vi "UHR-Fleezers Control (host) - Lorentz v2.vi"() -> ()   [LabVIEW 2014] (continued)
            n2219 = Build Cluster Array(w3307, w3324, w3323, w3322) -> (w3321:T46)
            n2220 = for {
              tunnel: w3343 -> [w3354]
              tunnel: w3321 -> [w3355] mode=indexing
              shift-right: [w3352] -> w3319
              shift-left: TRUE -> [w3353]
              shift-right: [w3351] -> w3317
              shift-left: _ -> [w3347]
              shift-right: [w3350] -> w3316
              shift-left: _ -> [w3346]
              shift-right: [w3349] -> w3315
              shift-left: _ -> [w3345]
              shift-right: [w3348] -> w3314
              shift-left: _ -> [w3344]
              n2221 = case shown="True" w3353 {
                selector: w3353 -> [w3360 _]
                tunnel: w3355 -> [_ w3369]
                tunnel: w3354 -> [_ w3367]
                tunnel: [w3360 w3365] -> w3352
                tunnel: [w3359 w3364] -> w3351
                tunnel: [w3358 w3363] -> w3350
                tunnel: [w3357 w3362] -> w3349
                tunnel: [w3356 w3361] -> w3348
                tunnel: w3347 -> [w3359 _]
                tunnel: w3346 -> [w3358 _]
                tunnel: w3345 -> [w3357 _]
                tunnel: w3344 -> [w3356 _]
                frame False {
                }
                frame True {
                  n2222 = Unbundle(w3369) -> (w3368:T45)
                  n2223 = call "isclickinwindow.vi"("Image Param"=w3368, "Point32"=w3367) -> ("4 Y"=w3361:i32, "3 Height"=w3362:i32, "2 X"=w3363:i32, "1 Width"=w3364:i32, "In image?"=w3366:bool)  [unwired: 1 in]
                  n2224 = Not(x=w3366) -> (.not. x?=w3365:bool)
                }
              }
            }
            n2225 = Not(x=w3319) -> (.not. x?=w3318:bool)
            n2226 = case shown="True" w3318 {
              tunnel: w3316 -> [_ w3383]
              tunnel: w3314 -> [_ w3382]
              tunnel: w3317 -> [_ w3381]
              tunnel: w3315 -> [_ w3380]
              frame False {
              }
              frame True {
                w3370 = FALSE ("Get Point")
                n2227 = local read "Scan lines (y)"() -> (w3385:u64)
                n2228 = disable-structure shown="Disabled" {
                  frame Disabled {
                  }
                  frame Enabled {
                  }
                }
                n2229 = local read "Actual MCL Inc (V)"() -> (w3379:dbl)
                n2230 = local read "Scan steps (MCL)"() -> (w3384:u64)
                n2231 = Divide "Y Pix/step"(x=w3380, y=w3385) -> (x/y=w3392:dbl)
                n2232 = Divide "Y V/pix"(x=w3379, y=w3392) -> (x/y=w3391:dbl)
                n2233 = Divide "Y half step offset"(x=w3379, y=2.0) -> (x/y=w3393:dbl)
                n2234 = Divide "X pix/step"(x=w3381, y=w3384) -> (x/y=w3390:dbl)
                n2235 = Negate(x=w3393) -> (-x=w3394:dbl)
                n2236 = local read "Initial Y"() -> (w3400:dbl)
                n2237 = Multiply(x=w3382, y=w3391) -> (x*y=w3401:dbl)
                n2238 = Divide "X half step offset"(x=w3379, y=2.0) -> (x/y=w3387:dbl)
                n2239 = Divide "X V/pix"(x=w3379, y=w3390) -> (x/y=w3389:dbl)
                n2240 = Multiply(x=w3379, y=w3384) -> (x*y=w3396:dbl)
                n2241 = Compound Arithmetic op=ADD(w3394, w3401, w3400) -> (w3371:dbl)
                "Pointer Y (V)" <- w3371
                n2242 = Multiply(x=w3389, y=w3383) -> (x*y=w3398:dbl)
                n2243 = Negate(x=w3387) -> (-x=w3386:dbl)
                n2244 = local read "Initial X"() -> (w3399:dbl)
                n2245 = Negate(x=w3398) -> (-x=w3397:dbl)
                n2246 = Compound Arithmetic op=ADD(w3386, w3396, w3399, w3397) -> (w3372:dbl)
                "Pointer X (V)" <- w3372
                n2247 = case shown="True" "Set High F Confocal Spot (X-Y)" {
                  tunnel: w3372 -> [_ w3402]
                  tunnel: w3371 -> [_ w3403]
                  frame False {
                  }
                  frame True {
                    "Confocal Y 2 (V)" <- w3403
                    "Confocal X 2 (V)" <- w3402
                  }
                }
                n2248 = Or(x="Set X Only", y="Set Confocal Spot (X-Y)") -> (x .or. y?=w3375:bool)
                n2249 = Or(x="Set Confocal Spot (X-Y)", y="Set Y Only") -> (x .or. y?=w3374:bool)
                n2250 = case shown="True" w3375 {
                  tunnel: w3372 -> [_ w3404]
                  frame False {
                  }
                  frame True {
                    n2251 = property on="AO2" class="Slide (strict)"("Val(Sgnl)"=w3404) -> ()  [unwired: 2 in, 2 out]
                    "Confocal X 1 (V)" <- w3404
                  }
                }
                n2252 = case shown="True" w3374 {
                  tunnel: w3371 -> [_ w3405]
                  frame False {
                  }
                  frame True {
                    n2253 = property on="AO1" class="Slide (strict)"("Val(Sgnl)"=w3405) -> ()  [unwired: 2 in, 2 out]
                    "Confocal Y 1 (V)" <- w3405
                  }
                }
                n2254 = local write "Set High F Confocal Spot (X-Y)"(w3370) -> ()
                n2255 = local write "Set Confocal Spot (X-Y)"(w3370) -> ()
                n2256 = local write "Set X Only"(w3370) -> ()
                n2257 = local write "Set Y Only"(w3370) -> ()
              }
            }
          }
          frame 3 {
            n2258 = local read "BD 2 Frequency 1 (MHz)"() -> (w3407:dbl)
            n2259 = local read "BD 1 Frequency 1 (MHz)"() -> (w3408:dbl)
            n2260 = local write "Manipulating Trap"(TRUE ("Manipulating Trap")) -> ()
            n2261 = local write "Coords"(T9 {"Horizontal"=0, "Vertical"=0} ("Coords")) -> ()
            n2262 = while {
              tunnel: w3412 -> [w3417]
              tunnel: w3410 -> [w3416]
              tunnel: w3408 -> [w3415]
              tunnel: w3407 -> [w3414]
              tunnel: w3406 -> [w3413]
              stop <- w3418 stop-if-true
              n2263 = event shown="[0] \"Pane\": Mouse Move" {
                selector: _ -> [_ _]
                dyn-events: _ -> [_ _]
                timeout: _ -> [_ _]
                tunnel: ["Force Manip Abort" w3482] -> w3418
                tunnel: w3417 -> [w3425 _]
                tunnel: w3416 -> [w3423 _]
                tunnel: w3415 -> [w3422 _]
                tunnel: w3414 -> [w3421 _]
                tunnel: w3413 -> [w3419 _]
                event Mouse Move {
                  n2264 = event-data() -> ("Time"=w3426:u32, "Coords"=w3427:T9)  [unwired: 3 out]
                  n2265 = Less?(x=w3426, y=w3425) -> (x < y?=w3424:bool)
                  n2266 = case "Makes sure old motion events prior to mouse click aren't used" shown="False" w3424 {
                    tunnel: w3427 -> [w3469 _]
                    tunnel: w3423 -> [w3470 _]
                    tunnel: w3422 -> [w3444 _]
                    tunnel: w3421 -> [w3443 _]
                    tunnel: w3419 -> [w3428 _]
                    frame False {
                      n2267 = Subtract(x=w3469, y=w3470) -> (x-y=w3468:T9)
                      "Coords" <- w3468
                      n2268 = local read "Y RF Frequency Limits (MHz)"() -> (w3429:T20)
                      n2269 = To Double Precision Float(number=w3468) -> (double precision float=w3467:cluster{"Horizontal":dbl, "Vertical":dbl})
                      n2270 = Multiply(x=cluster{"Horizontal":dbl, "Vertical":dbl} {"Horizontal"=-1.0, "Vertical"=1.0}, y="Manipulation Scaling") -> (x*y=w3463:cluster{"Horizontal":dbl, "Vertical":dbl})
                      n2271 = local read "X RF Frequency Limits (MHz)"() -> (w3430:T20)
                      n2272 = Multiply(x=w3467, y=w3463) -> (x*y=w3465:cluster{"Horizontal":dbl, "Vertical":dbl})
                      n2273 = Unbundle By Name(w3465) -> ("Horizontal"=w3460:dbl, "Vertical"=w3464:dbl)
                      n2274 = Unbundle By Name(w3429) -> ("Maximum"=w3432:dbl, "Minimum"=w3431:dbl)
                      n2275 = Boolean To (0,1)(Boolean="Manip. X?") -> (0, 1=w3458:i16)
                      n2276 = Boolean To (0,1)(Boolean="Manip. Y?") -> (0, 1=w3455:i16)
                      n2277 = local read "BD 1 Frequency 2 (MHz)"() -> (w3446:dbl)
                      n2278 = Multiply(x=w3464, y=w3455) -> (x*y=w3457:dbl)
                      n2279 = Multiply(x=w3458, y=w3460) -> (x*y=w3461:dbl)
                      n2280 = local read "BD 2 Frequency 2 (MHz)"() -> (w3445:dbl)
                      n2281 = Unbundle By Name(w3430) -> ("Maximum"=w3434:dbl, "Minimum"=w3433:dbl)
                      n2282 = Add(x=w3443, y=w3457) -> (x+y=w3436:dbl)
                      n2283 = Add(x=w3444, y=w3461) -> (x+y=w3438:dbl)
                      n2284 = In Range and Coerce(upper limit=w3434, x=w3438, lower limit=w3433) -> (coerced(x)=w3437:dbl)  [unwired: 1 out]
                      n2285 = In Range and Coerce(upper limit=w3432, x=w3436, lower limit=w3431) -> (coerced(x)=w3435:dbl)  [unwired: 1 out]
                      n2286 = Subtract(x=w3437, y=w3446) -> (x-y=w3454:dbl)
                      n2287 = Subtract(x=w3435, y=w3445) -> (x-y=w3453:dbl)
                      n2288 = Square(x=w3454) -> (x^2=w3452:dbl)
                      n2289 = Square(x=w3453) -> (x^2=w3451:dbl)
                      n2290 = Add(x=w3452, y=w3451) -> (x+y=w3450:dbl)
                      n2291 = Square Root(x=w3450) -> (sqrt(x)=w3447:dbl)
                      n2292 = In Range and Coerce(upper limit="Limit Max (MHz)", x=w3447, lower limit="Limit Min (MHz)") -> (In Range?=w3440:bool)  [unwired: 1 out]
                      n2293 = Not(x="Limits Enable") -> (.not. x?=w3439:bool)
                      n2294 = Or(x=w3440, y=w3439) -> (x .or. y?=w3441:bool)
                      n2295 = case shown="True" w3441 {
                        tunnel: w3447 -> [_ w3472]
                        tunnel: w3437 -> [_ w3479]
                        tunnel: w3446 -> [_ w3478]
                        tunnel: w3435 -> [_ w3477]
                        tunnel: w3445 -> [_ w3476]
                        tunnel: w3430 -> [_ w3474]
                        tunnel: w3429 -> [_ w3473]
                        tunnel: w3428 -> [_ w3471]
                        frame False {
                        }
                        frame True {
                          n2296 = local read "BD 1 Frequency 3 (MHz)"() -> (w3480:dbl)
                          n2297 = local read "BD 2 Frequency 3 (MHz)"() -> (w3475:dbl)
                          n2298 = local write "Trap Delta (MHz)"(w3472) -> ()
                          n2299 = call "set RF board frequency - interlace.vi"("Board 2 Frequency Limits"=w3473, "Board 1 Frequency Limits"=w3474, "FPGA VI Reference In"=w3471, "Board 2 Frequency 3 (MHz)"=w3475, "Board 1 Frequency 3 (MHz)"=w3480, "Board 2 Frequency 2 (MHz)"=w3476, "Board 2 Frequency 1 (MHz)"=w3477, "Board 1 Frequency 2 (MHz)"=w3478, "Board 1 Frequency 1  (MHz)"=w3479) -> ()  [unwired: 1 in, 2 out]
                          n2300 = local write "BD 2 Frequency 1 (MHz)"(w3477) -> ()
                          n2301 = local write "BD 1 Frequency 1 (MHz)"(w3479) -> ()
                        }
                      }
                    }
                    frame True {
                    }
                  }
                }
                event Mouse Up {
                  n2302 = event-data() -> ("Button"=w3481:u16)  [unwired: 8 out]
                  n2303 = case shown="3" w3481 {
                    tunnel: [FALSE TRUE] -> w3482
                    frame 0, Default {
                    }
                    frame 3 {
                      n2304 = local read "Trap Delta (MHz)"() -> (w3484:dbl)
                      n2305 = property on="Initial delta (MHz)" class="DigNum (strict)"("Val(Sgnl)"=w3484) -> ()  [unwired: 2 in, 2 out]
                      n2306 = local write "Manipulating Trap"(FALSE ("Manipulating Trap")) -> ()
                    }
                  }
                }
              }
            }
          }
        }
      }
      event Timeout {
        n2307 = event-data() -> ()  [unwired: 4 out]
      }
      event "Stop All": Mouse Down {
        n2308 = event-data() -> ()  [unwired: 9 out]
      }
      event Mouse Move {
        n2309 = event-data() -> ()  [unwired: 6 out]
      }
    }
    n2310 = node-c288() -> ()  [unwired: 2 out]
  }
  n2311 = disable-structure shown="Disabled" {
    frame Disabled {
      n2312 = flat-sequence "Video" {
        tunnel: [w3499] -> w3488
        tunnel: w3488 -> [w3540]
        frame #0 {
          w3489 = FALSE ("File open?")
          n2313 = while {
            stop <- w3491 continue-if-true
            n2314 = call "Close Video Capture.vi"() -> ("error code OUT"=w3493:i32)
            n2315 = Equal?(x=w3493, y=0) -> (x = y?=w3491:bool)
          }
          n2316 = local write "New Video File"(w3489) -> ()
          n2317 = local write "File open?"(w3489) -> ()
          n2318 = local write "Save Video"(w3489) -> ()
          n2319 = local write "Stop All"(FALSE ("Stop All")) -> ()
        }
        frame #1 {
          n2320 = call "DMR_Init.vi"() -> ()  [unwired: 3 out]
        }
        frame #2 {
          w3494 = "DE245428202"  # MSU fleezers card #
          (unwired) "DE019116701"  # Illinois fleezers card #
          # "Setting the destination format to Mono8 makes sure that the image can be displayed in the intensity plot."
          n2321 = call "DMR_GetDevice.vi"("search string IN"=w3494) -> ("device handle OUT"=w3517:i32)  [unwired: 4 in, 2 out]
          n2322 = call "DMR_OpenDevice.vi"("device handle IN"=w3517) -> ("driver handle OUT"=w3500:i32)  [unwired: 4 out]
          n2323 = call "DMR_FindList.vi"("flags IN"=u32 0 ("flags"), "list name IN"="" ("String"), "list type IN"=T47."camera descriptions", "driver handle IN"=w3500) -> ("list handle OUT"=w3503:i32)  [unwired: 2 out]
          n2324 = call "DMR_FindList.vi"("flags IN"=u32 0 ("flags"), "list name IN"="Base", "list type IN"=T47."setting", "driver handle IN"=w3500) -> ("list handle OUT"=w3501:i32)  [unwired: 2 out]
          n2325 = call "OBJ_GetHandle.vi"("object name IN"="VideoStandard", "list handle IN"=w3503) -> ("object handle OUT"=w3497:i32)  [unwired: 3 out]
          n2326 = call "OBJ_GetHandle.vi"("object name IN"="PixelFormat", "list handle IN"=w3501) -> ("object handle OUT"=w3511:i32)  [unwired: 3 out]
          n2327 = call "OBJ_SetS.vi"("value index IN"=0, "value IN"="NTSC M", "object handle IN"=w3497) -> ()  [unwired: 2 out]
          n2328 = call "OBJ_SetS.vi"("value index IN"=0, "value IN"="Mono8" ("value"), "object handle IN"=w3511) -> ()  [unwired: 2 out]
          n2329 = call "OBJ_GetHandle.vi"("object name IN"="VideoChannel", "list handle IN"=w3501) -> ("object handle OUT"=w3507:i32)  [unwired: 3 out]
          n2330 = while {
            tunnel: [w3521] -> w3499
            tunnel: w3500 -> [w3518]
            stop <- w3519 continue-if-true
            n2331 = call "DMR_ImageRequestSingle.vi"("request control IN"=0, "driver handle IN"=w3518) -> ("error code OUT"=w3520:i32, "driver handle OUT"=w3521:i32)  [unwired: 2 out]
            n2332 = Equal To 0?(x=w3520) -> (x = 0?=w3519:bool)
          }
          n2333 = call "OBJ_SetI.vi"("value index IN"=0, "value IN"="Video channel", "object handle IN"=w3507) -> ()  [unwired: 2 out]
        }
        frame #3 {
          w3528 = T25 0 items=["Grayscale (U8)", "Grayscale (I16)", "Grayscale (SGL)", "Complex (CSG)", "RGB (U32)", "HSL (U32)", "RGB (U64)"] ("Image Type")
          w3536 = T25 0 items=["Grayscale (U8)", "Grayscale (I16)", "Grayscale (SGL)", "Complex (CSG)", "RGB (U32)", "HSL (U32)", "RGB (U64)"] ("Image Type")
          n2334 = call "IMAQ AVI2 Get Codec Names"() -> ("Codec Names"=w3523:string[])  [unwired: 10 in, 1 out]
          "Installed Codec Names" <- w3523
          n2335 = for "Create Greyscale map" {
            N: 256 -> [_]
            tunnel: [w3542] -> w3525 mode=indexing
            workers-P: _ -> [_]
            i -> [w3545]
            n2336 = To Unsigned Byte Integer(number=w3545) -> (unsigned 8bit integer=w3541:u8)
            n2337 = Join Numbers(hi=w3541, lo=w3541) -> ((hi.lo)=w3544:u16)
            n2338 = Join Numbers(hi=w3541, lo=w3541) -> ((hi.lo)=w3543:u16)
            n2339 = Join Numbers(hi=w3544, lo=w3543) -> ((hi.lo)=w3542:u32)
          }
          n2340 = property on="Codec choice" class="CmbBox"("Strings[]"=w3523) -> ()  [unwired: 2 in, 2 out]
          n2341 = call "IMAQ Create"("Image Name"="Scaled video", "Image Type"=w3528) -> ("New Image"=w3527:T2)  [unwired: 2 in, 2 out]
          n2342 = call "IMAQ Create"("Image Name"="Main video", "Image Type"=w3536) -> ("New Image"=w3537:T2)  [unwired: 2 in, 2 out]
          n2343 = node-c288(0 ("Processor")) -> (w3535:T35)  [unwired: 3 out]
          n2344 = Initialize Array(u32 0 ("Window Number (0...15)"), 480 ("dimension size"), 640 ("dimension size")) -> (w3530:u32[][])
          n2345 = timed-loop {
            tunnel: w3540 -> [w3562]
            tunnel: [w3561] -> w3539
            tunnel: w3537 -> [w3560]
            timing: w3535 -> [_]
            timing-out: [_] -> w3534
            tunnel: w3530 -> [w3553]
            tunnel: w3527 -> [w3551]
            tunnel: w3525 -> [w3550]
            stop <- w3552 stop-if-true
            # "This block performs the \nactual image capture."
            n2346 = node-c288() -> (→"Finished Late? [i-1]":bool)  [unwired: 5 out]
            n2347 = local read "Stop All"() -> (w3552:bool)
            n2348 = feedback #1(T48 refnum ("AVI Refnum")) -> (w3558:T48)
            n2349 = case shown="True" "New Video File" {
              tunnel: [w3575 w3576] -> w3549
              tunnel: w3558 -> [w3575 w3577]
              frame False {
              }
              frame True {
                n2350 = flat-sequence {
                  tunnel: w3577 -> [w3579]
                  tunnel: [w3581] -> w3576
                  frame #0 {
                    n2351 = local read "File open?"() -> (w3578:bool)
                    n2352 = case shown="True" w3578 {
                      tunnel: w3579 -> [_ w3580]
                      frame False {
                      }
                      frame True {
                        n2353 = call "IMAQ AVI2 Close"("AVI Refnum"=w3580) -> ()  [unwired: 10 in, 1 out]
                      }
                    }
                  }
                  frame #1 {
                    n2354 = local write "New Video File"(FALSE ("New Video File")) -> ()
                    n2355 = call "Create new save file.vi"("Ext"=".avi" ("string"), "Index In"="Video Index") -> ("Path Out"=w3584:path, "Index Out"=w3586:dbl)  [unwired: 1 in]
                    "Path Out" <- w3584
                    n2356 = local write "Video Index"(w3586) -> ()
                    n2357 = call "IMAQ AVI2 Create"("Codec"="Codec choice", "Frames Per Second"=u32 30, "AVI Path"=w3584) -> ("AVI Refnum"=w3581:T48)  [unwired: 7 in, 1 out]
                    "File open?" <- TRUE ("Files open?")
                  }
                }
              }
            }
            n2358 = feedback-in #1(w3549) -> ()
            n2359 = call "DMR_ImageRequestWaitFor.vi"("queue number IN"=0, "timeout(ms) IN"=500, "driver handle IN"=w3562) -> ("error code OUT"=w3566:i32, "request number OUT"=w3563:i32, "driver handle OUT"=w3564:i32)
            n2360 = Equal To 0?(x=w3566) -> (x = 0?=w3565:bool)
            n2361 = Reciprocal(x="Video Capture Rate (Hz)") -> (1/x=w3556:dbl)
            n2362 = Multiply(x=w3556, y=1000.0) -> (x*y=w3554:dbl)
            n2363 = case shown="True" w3565 {
              tunnel: w3564 -> [w3590 w3627]
              tunnel: w3563 -> [_ w3626]
              tunnel: [w3590 w3623] -> w3561
              tunnel: w3560 -> [_ w3609]
              tunnel: w3553 -> [_ w3612]
              tunnel: w3549 -> [_ w3592]
              tunnel: w3551 -> [_ w3606]
              tunnel: w3550 -> [_ w3605]
              frame False {
              }
              frame True {
                w3617 = u32 0 ("X-offset IN")
                n2364 = call "DMR_GetImageRequestBufferData.vi"("driver handle IN"=w3627, "request number IN"=w3626) -> ("width OUT"=w3616:i32, "height OUT"=w3615:i32, "driver handle OUT"=w3622:i32, "request number OUT"=w3621:i32, "bytes per pixel OUT"=w3618:i32)  [unwired: 13 out]
                n2365 = call "DMR_GetImageRequestBufferImageData.vi"("driver handle IN"=w3622, "request number IN"=w3621, "bytes per pixel IN"=w3618, "X-offset IN"=w3617, "Y-offset IN"=w3617, "height IN"=w3615, "width IN"=w3616) -> ("driver handle OUT"=w3620:u32, "request number OUT"=w3619:u32, "image OUT"=w3598:u32[][])  [unwired: 10 out]
                n2366 = Transpose 2D Array(2D array=w3598) -> (transposed array=w3604:u32[][])
                n2367 = Select(t=w3604, s="Flip Y (or X)", f=w3598) -> (s? t:f=w3603:u32[][])
                n2368 = call "DMR_ImageRequestUnlock.vi"("request number IN"=w3619, "driver handle IN"=w3620) -> ("driver handle OUT"=w3625:i32)  [unwired: 1 in, 2 out]
                n2369 = for {
                  tunnel: w3603 -> [w3662] mode=indexing
                  tunnel: [w3661] -> w3601 mode=indexing
                  n2370 = Reverse 1D Array(array=w3662) -> (reversed array=w3661:u32[])
                }
                n2371 = call "DMR_ImageRequestSingle.vi"("request control IN"=0, "driver handle IN"=w3625) -> ("driver handle OUT"=w3623:i32)  [unwired: 3 out]
                n2372 = Transpose 2D Array(2D array=w3601) -> (transposed array=w3602:u32[][])
                n2373 = Select(t=w3602, s="Flip Y (or X)", f=w3601) -> (s? t:f=w3599:u32[][])
                n2374 = Select(t=w3599, s="Flip Image", f=w3598) -> (s? t:f=w3596:u32[][])
                n2375 = case shown="True" "Averaging" {
                  tunnel: w3596 -> [w3673 w3678]
                  tunnel: [w3673 w3677] -> w3610
                  tunnel: w3612 -> [_ w3675]
                  frame False {
                  }
                  frame True {
                    (unwired) 1
                    w3683 = 1
                    n2376 = feedback #2(w3675) -> (w3674:u32[][])
                    n2377 = Add(x=w3678, y=w3674) -> (x+y=w3679:u32[][])
                    n2378 = Select(t=w3675, s="Reset Averaging", f=w3679) -> (s? t:f=w3681:u32[][])
                    n2379 = feedback-in #2(w3681) -> ()
                    n2380 = feedback #3(w3683) -> (w3676:i32)
                    n2381 = Divide(x=w3679, y=w3676) -> (x/y=w3680:dbl[][])
                    n2382 = Increment(x=w3676) -> (x+1=w3684:i32)
                    n2383 = To Unsigned Long Integer(number=w3680) -> (unsigned 32bit integer=w3677:u32[][])
                    n2384 = Select(t=w3683, s="Reset Averaging", f=w3684) -> (s? t:f=w3682:i32)
                    n2385 = feedback-in #3(w3682) -> ()
                  }
                }
                n2386 = case shown="True" "Zoom video window" {
                  tunnel: w3610 -> [_ w3641]
                  tunnel: w3606 -> [_ w3640]
                  frame False {
                  }
                  frame True {
                    n2387 = To Double Precision Float(number=w3641) -> (double precision float=w3638:dbl[][])
                    n2388 = In Range and Coerce(upper limit="Intensity Upper", x=w3638, lower limit="Intensity Lower") -> (coerced(x)=w3637:dbl[][])  [unwired: 1 out]
                    n2389 = Subtract(x="Intensity Upper", y="Intensity Lower") -> (x-y=w3634:dbl)
                    n2390 = Subtract(x=w3637, y="Intensity Lower") -> (x-y=w3635:dbl[][])
                    n2391 = Divide(x=w3635, y=w3634) -> (x/y=w3636:dbl[][])
                    n2392 = Multiply(x=255.0, y=w3636) -> (x*y=w3632:dbl[][])
                    n2393 = To Unsigned Byte Integer(number=w3632) -> (unsigned 8bit integer=w3639:u8[][])
                    n2394 = call "IMAQ ArrayToImage"("Image Pixels (U8)"=w3639, "Image"=w3640) -> ("Image Out"=w3628:T2)  [unwired: 4 in, 5 out]
                    n2395 = First Call?() -> (First Call?: T/F=w3629:bool)
                    n2396 = case shown="True" w3629 {
                      tunnel: w3628 -> [w3642 w3653]
                      frame False {
                        n2397 = flat-sequence {
                          tunnel: w3642 -> [w3648]
                          frame #0 {
                            w3645 = FALSE ("Get/Set Status? (Set)")
                            w3644 = 0 ("Window Number (0...15)")
                            n2398 = call "IMAQ WindSize"("Get/Set Status? (Set)"=w3645, "Window Number"=w3644) -> ("Width & Height out"=→"Window Size":cluster{"Width":i32, "Height":i32})  [unwired: 4 in, 2 out]
                            n2399 = call "IMAQ WindMove"("Window Number (0...15)"=w3644, "Get/Set Status? (Set)"=w3645) -> ("Coordinates (screen)"=→"Window Position":cluster{"X Position":i32, "Y Position":i32})  [unwired: 3 in, 1 out]
                            n2400 = call "IMAQ WindDraw"("Resize to Image Size? (Y)"=FALSE, "Window Number (0...15)"=w3644, "Image"=w3648) -> ()  [unwired: 7 in, 2 out]
                          }
                          frame #1 {
                            n2401 = call "IMAQ WindZoom 2"("Center Point"="Center Point", "Zoom to Fit? (False)"=FALSE, "Zoom Factor"="Zoom Factor") -> ()  [unwired: 5 in, 4 out]
                          }
                        }
                      }
                      frame True {
                        n2402 = flat-sequence {
                          tunnel: w3653 -> [w3656]
                          tunnel: [w3654] -> w3652
                          tunnel: w3652 -> [w3658]
                          frame #0 {
                            w3655 = TRUE ("Resize to Image Size? (Y)")
                            w3654 = 0 ("Window Number (0...15)")
                            n2403 = call "IMAQ WindNonTearing"("Window Number"=w3654, "NonTearing? (True)"=w3655) -> ()  [unwired: 8 in, 2 out]
                            n2404 = call "IMAQ WindDraw"("Resize to Image Size? (Y)"=w3655, "Window Number (0...15)"=w3654, "Image"=w3656) -> ()  [unwired: 7 in, 2 out]
                          }
                          frame #1 {
                            n2405 = call "IMAQ WindSize"("Scrollbars? (N)"=FALSE, "Width & Height"="Initial Window Size", "Window Number"=w3658) -> ()  [unwired: 3 in, 3 out]
                            n2406 = call "IMAQ WindMove"("Window Number (0...15)"=w3658, "Coordinates (screen)"="Initial Window Position") -> ()  [unwired: 3 in, 2 out]
                          }
                        }
                      }
                    }
                  }
                }
                n2407 = To Unsigned Byte Integer(number=w3610) -> (unsigned 8bit integer=w3608:u8[][])
                n2408 = call "IMAQ ArrayToImage"("Image Pixels (U8)"=w3608, "Image"=w3609) -> ("Image Out"=w3607:T2)  [unwired: 4 in, 5 out]
                "Primary Video Display" <- w3607
                n2409 = Not(x="Close Video File") -> (.not. x?=w3594:bool)
                n2410 = And(x="Save Video", y=w3594) -> (x .and. y?=w3591:bool)
                n2411 = case shown="True" "Save Image" {
                  tunnel: w3608 -> [_ w3687]
                  tunnel: w3605 -> [_ w3686]
                  frame False {
                  }
                  frame True {
                    n2412 = call <vilib>:"Flatten Pixmap.vi"("colors"=w3686, "8-bit pixmap"=w3687) -> ("image data"=w3693:T49)  [unwired: 4 in, 5 out]
                    n2413 = call "Create new save file.vi"("Insert"="video_frame_" ("string"), "Ext"=".bmp" ("string"), "Index In"="Image Index") -> ("Path Out"=w3689:path, "Index Out"=w3694:dbl)
                    n2414 = Increment(x=w3694) -> (x+1=w3688:dbl)
                    n2415 = local write "Image Index"(w3688) -> ()
                    n2416 = call <vilib>:"Write BMP File.vi"("image data"=w3693, "path to BMP file"=w3689) -> ()  [unwired: 1 in, 9 out]
                  }
                }
                n2417 = case shown="True" w3591 {
                  tunnel: w3592 -> [w3664 w3669]
                  tunnel: w3607 -> [_ w3668]
                  tunnel: "Close Video File" -> [w3663 _]
                  frame False {
                    n2418 = case shown="True" w3663 {
                      tunnel: w3664 -> [_ w3665]
                      frame False {
                      }
                      frame True {
                        w3666 = FALSE ("Save Video")
                        n2419 = call "IMAQ AVI2 Close"("AVI Refnum"=w3665) -> ()  [unwired: 10 in, 1 out]
                        n2420 = local write "File open?"(w3666) -> ()
                        n2421 = local write "Save Video"(w3666) -> ()
                      }
                    }
                  }
                  frame True {
                    n2422 = local read "File open?"() -> (w3667:bool)
                    n2423 = case shown="True" w3667 {
                      tunnel: w3669 -> [_ w3672]
                      tunnel: w3668 -> [_ w3671]
                      frame False {
                        n2424 = local write "New Video File"(TRUE ("New Video File")) -> ()
                      }
                      frame True {
                        n2425 = call "IMAQ AVI2 Write Frame"("Image"=w3671, "AVI Refnum"=w3672) -> ()  [unwired: 7 in, 3 out]
                      }
                    }
                  }
                }
              }
            }
            n2426 = node-c288(w3554, "Deadline (ms)") -> ()  [unwired: 1 out]
          }
          n2427 = node-c288(w3534) -> ()  [unwired: 1 out]
          n2428 = call "DMR_CloseDevice.vi"("driver handle IN"=w3539) -> ()  [unwired: 1 in, 4 out]
        }
        frame #4 {
          n2429 = call "DMR_Close.vi"() -> ()  [unwired: 1 out]
        }
      }
    }
    frame Enabled {
    }
  }
  n2430 = node-c288(3 ("Processor")) -> (w60:T35)  [unwired: 3 out]
  n2431 = timed-loop "Oscillate Trap/AOM (fishing, conjugate plane alignment)" {
    tunnel: [w3701] -> w65
    timing: w60 -> [_]
    timing-out: [_] -> w59
    tunnel: w21 -> [w3700]
    tunnel: w9 -> [w3699]
    stop <- w3701 stop-if-true
    n2432 = node-c288() -> ()  [unwired: 2 out]
    n2433 = event shown="[1] \"Fl. Triggered...\": Value Change" {
      selector: _ -> [_ _ _ _]
      dyn-events: _ -> [_ _ _ _]
      timeout: _ -> [_ _ _ _]
      tunnel: [FALSE ("Stop All") _ _ w4372] -> w3701
      tunnel: w3700 -> [w3704 _ _ _]
      tunnel: w3699 -> [_ _ w4309 _]
      event "Oscillate Set 1", "Fish for Tether": Value Change {
        n2434 = event-data() -> ()  [unwired: 6 out]
        n2435 = local read "Oscillate Set 1"() -> (w3708:bool)
        n2436 = Or(x=w3708, y="Fish for Tether") -> (x .or. y?=w3706:bool)
        n2437 = case shown="True" w3706 {
          tunnel: "Fish for Tether" -> [_ w3711]
          tunnel: w3704 -> [_ w3709]
          frame False {
          }
          frame True {
            n2438 = case shown="True" w3711 {
              selector: w3711 -> [w3714 w3720]
              tunnel: [w3714 w3720] -> w3710
              frame False {
              }
              frame True {
                n2439 = local write "Scan axis 2"(TRUE) -> ()
                n2440 = local write "Tether"(FALSE ("Tether")) -> ()
                n2441 = local read "Flow ON during cal?"() -> (w3715:bool)
                n2442 = property on="Trap Delta (MHz)" class="DigNum (strict)"("Val(Sgnl)"="Furthest Delta (MHz)") -> ()  [unwired: 2 in, 2 out]
                n2443 = Or(x="Flow ON during \nfishing?", y=w3715) -> (x .or. y?=w3716:bool)
                n2444 = Wait (ms)(milliseconds to wait=u32 500) -> ()  [unwired: 1 out]
                n2445 = property on="Sample Channel\nFlow" class="Bool (strict)"("Val(Sgnl)"=w3716) -> ()  [unwired: 2 in, 2 out]
              }
            }
            n2446 = node-c288() -> (w3713:T35)  [unwired: 1 in, 3 out]
            n2447 = timed-loop "Oscillate AOD" {
              timing: w3713 -> [_]
              timing-out: [_] -> w3712
              tunnel: w3710 -> [w3724]
              tunnel: w3709 -> [w3723]
              i -> [w3732]
              stop <- w3730 stop-if-true
              n2448 = node-c288() -> (w3731:i64)  [unwired: 1 out]
              n2449 = flat-sequence {
                tunnel: w3732 -> [w3759]
                tunnel: w3731 -> [w3758]
                tunnel: w3724 -> [w3742]
                tunnel: [w3742] -> w3729
                tunnel: [w3741] -> w3728
                tunnel: [w3740] -> w3727
                tunnel: [w3737] -> w3725
                tunnel: w3723 -> [w3733]
                tunnel: w3729 -> [w3806]
                tunnel: w3728 -> [w3804]
                tunnel: w3727 -> [w3803]
                tunnel: [w3802] -> w3726
                tunnel: w3725 -> [w3801]
                tunnel: [w3878] -> w3730
                tunnel: w3726 -> [w3877]
                frame #0 {
                  # "w (rad/s)"
                  # "t (s)"
                  n2450 = Divide(x=w3758, y=i64 1000) -> (x/y=w3734:dbl)
                  n2451 = local read "BD 1 Frequency 2 (MHz)"() -> (w3736:dbl)
                  n2452 = Multiply(x="Osc. freq. (Hz)", y=6.283185307179586) -> (x*y=w3756:dbl)
                  n2453 = Multiply(x=w3734, y=w3759) -> (x*y=w3755:dbl)
                  n2454 = Multiply(x=w3756, y=w3755) -> (x*y=w3739:dbl)
                  n2455 = local read "BD 1 Frequency 1 (MHz)"() -> (w3744:dbl)
                  n2456 = case shown="True" w3742 {
                    tunnel: w3739 -> [w3765 w3784]
                    tunnel: w3744 -> [_ w3792]
                    tunnel: w3736 -> [_ w3793]
                    tunnel: [w3762 w3788] -> w3735
                    tunnel: [FALSE w3766] -> w3740
                    tunnel: [0.0 w3780] -> w3737
                    frame False {
                      n2457 = Sine(x=w3765) -> (sin(x)=w3763:dbl)
                      n2458 = Multiply(x=w3763, y="Osc. amp. (MHz)") -> (x*y=w3762:dbl)
                    }
                    frame True {
                      # "trap position goes from 0 to 1 (0 is when it is furthest away, 1 is when closest)\nso we want to test for tether only when farther away, or x < 1"
                      # "quit if taking too long"
                      # "oscillate the trap"
                      # "Test for tether"
                      n2459 = local read "Vec Mean of T1 T2"() -> (w3769:dbl[])
                      "Trigger Signal" <- w3769
                      n2460 = Cosine(x=w3784) -> (cos(x)=w3796:dbl)
                      n2461 = Subtract(x=w3793, y=w3792) -> (x-y=w3791:dbl)
                      n2462 = Decrement(x=w3796) -> (x-1=w3795:dbl)
                      n2463 = Subtract(x=w3791, y="Closest Delta (MHz)") -> (x-y=w3789:dbl)
                      n2464 = Divide(x=w3795, y=-2.0) -> (x/y=w3779:dbl)
                      n2465 = Greater?(x=w3769, y="Stop F (pN)") -> (0:w3786:bool[])
                      n2466 = Multiply(x=w3779, y=w3789) -> (x*y=w3788:dbl)
                      n2467 = Less?(x=w3779, y="Fish mask thresh") -> (x < y?=w3778:bool)
                      n2468 = Boolean To (0,1)(Boolean=w3778) -> (0, 1=w3776:i16)
                      n2469 = Multiply(x=w3776, y=w3769) -> (x*y=w3775:dbl[])
                      n2470 = Divide(x=w3784, y=6.283185307179586) -> (x/y=w3783:dbl)
                      n2471 = Round Toward +Infinity(x=w3783) -> (ceil(x): smallest int >= x=w3780:dbl)
                      "Attempts" <- w3780
                      n2472 = Greater?(x=w3775, y="Stop F (pN) (mask)") -> (0:w3773:bool[])
                      n2473 = Or Array Elements(Boolean array=w3786) -> (logical OR=w3771:bool)
                      n2474 = Or Array Elements(Boolean array=w3773) -> (logical OR=w3770:bool)
                      n2475 = Greater?(x=w3780, y="Attempt Limit") -> (0:w3782:bool)
                      n2476 = case shown="True" w3782 {
                        frame False {
                        }
                        frame True {
                          n2477 = local write "Fish for Tether"(FALSE ("Fish for Tether")) -> ()
                          n2478 = call <vilib>:"Beep.vi"() -> ()  [unwired: 3 in, 9 out]
                          n2479 = local read "Messages"() -> (w3798:string)
                          n2480 = call "Update messages.vi"("Message to add"="Tether fishing timeout." ("Messages"), "Old message string"=w3798) -> ("New message string"=→"Messages":string)
                        }
                      }
                      n2481 = Select(t=w3771, s="Normal (on) or masked test (off)", f=w3770) -> (s? t:f=w3768:bool)
                      n2482 = And(x="Stop Fishing When Tether", y=w3768) -> (x .and. y?=w3766:bool)
                    }
                  }
                  n2483 = local read "BD 2 Frequency 1 (MHz)"() -> (w3743:dbl)
                  n2484 = Select(t=w3744, s="Scan axis 2", f=w3743) -> (s? t:f=w3747:dbl)
                  n2485 = Add(x=w3735, y=w3747) -> (x+y=w3741:dbl)
                  n2486 = Select(t=w3741, s="Scan axis 2", f=w3744) -> (s? t:f=w3750:dbl)
                  n2487 = Select(t=w3743, s="Scan axis 2", f=w3741) -> (s? t:f=w3749:dbl)
                  n2488 = local read "BD 2 Frequency 2 (MHz)"() -> (w3752:dbl)
                  n2489 = local read "BD 2 Frequency 3 (MHz)"() -> (w3751:dbl)
                  n2490 = local read "Y RF Frequency Limits (MHz)"() -> (w3745:T20)
                  n2491 = local read "X RF Frequency Limits (MHz)"() -> (w3746:T20)
                  n2492 = local read "BD 1 Frequency 3 (MHz)"() -> (w3753:dbl)
                  n2493 = call "set RF board frequency - interlace.vi"("Board 2 Frequency Limits"=w3745, "Board 1 Frequency Limits"=w3746, "FPGA VI Reference In"=w3733, "Board 2 Frequency 3 (MHz)"=w3751, "Board 1 Frequency 3 (MHz)"=w3753, "Board 2 Frequency 2 (MHz)"=w3752, "Board 2 Frequency 1 (MHz)"=w3749, "Board 1 Frequency 2 (MHz)"=w3736, "Board 1 Frequency 1  (MHz)"=w3750) -> ()  [unwired: 1 in, 2 out]
                }
                frame #1 {
                  n2494 = And(x=w3806, y=w3803) -> (x .and. y?=w3805:bool)
                  n2495 = case "Only if were fishing and now formed tether" shown="True" w3805 {
                    tunnel: w3804 -> [w3808 w3823]
                    tunnel: [w3807 w3822] -> w3802
                    tunnel: w3801 -> [_ w3818]
                    frame False {
                      n2496 = local read "Fish for Tether"() -> (w3807:bool)
                      n2497 = case shown="False" w3807 {
                        tunnel: w3808 -> [w3809 _]
                        frame False {
                          n2498 = property on="BD 1 Frequency 1 (MHz)" class="DigNum (strict)"("Val(Sgnl)"=w3809) -> ()  [unwired: 2 in, 2 out]
                        }
                        frame True {
                        }
                      }
                    }
                    frame True {
                      w3822 = FALSE ("Fish for Tether")
                      n2499 = call <vilib>:"Beep.vi"() -> ()  [unwired: 3 in, 9 out]
                      n2500 = Number To Decimal String(number=w3818, width (-)=i16 1) -> (decimal integer string=w3816:string)
                      n2501 = Concatenate Strings("Formed tether in ", w3816, " attempt(s)." ("string")) -> (w3813:string)
                      n2502 = local read "Messages"() -> (w3820:string)
                      n2503 = local write "Fish for Tether"(w3822) -> ()
                      n2504 = call "Update messages.vi"("Message to add"=w3813, "Old message string"=w3820) -> ("New message string"=w3819:string)
                      n2505 = local write "Messages"(w3819) -> ()
                      n2506 = Get Date/Time In Seconds() -> (seconds since 1Jan1904=→"Time tether formed":timestamp)
                      n2507 = local read "Flow ON during cal?"() -> (w3810:bool)
                      n2508 = property on="Sample Channel\nFlow" class="Bool (strict)"("Val(Sgnl)"=w3810) -> (error out=w3811:errorcluster)  [unwired: 2 in, 1 out]
                      n2509 = case shown="\"2\", \"3\", \"4\", \"5\", \"6\"" "Then..." {
                        selector: "Then..." -> [_ w3826]
                        tunnel: w3823 -> [w3825 _]
                        tunnel: w3811 -> [_ _]
                        frame "1", Default {
                          n2510 = property on="BD 1 Frequency 1 (MHz)" class="DigNum (strict)"("Val(Sgnl)"=w3825) -> ()  [unwired: 2 in, 2 out]
                        }
                        frame "2", "3", "4", "5", "6" {
                          n2511 = flat-sequence {
                            tunnel: w3826 -> [w3828]
                            frame #0 {
                              n2512 = property on="Trap Delta (MHz)" class="DigNum (strict)"("Val(Sgnl)"="Move to Delta 1 (MHz)") -> ()  [unwired: 2 in, 2 out]
                            }
                            frame #1 {
                              n2513 = case shown="\"5\", \"6\"" w3828 {
                                selector: w3828 -> [w3831 w3841 _]
                                frame "3", "4" {
                                n2514 = flat-sequence {
                                tunnel: w3831 -> [w3832]
                                tunnel: [w3832] -> w3829
                                tunnel: [w3834] -> w3830
                                tunnel: w3829 -> [w3834]
                                tunnel: w3830 -> [w3838]
                                frame #0 {
                                n2515 = property on="Green Laser ON" class="Bool (strict)"("Val(Sgnl)"=TRUE ("Value (Signaling)")) -> ()  [unwired: 2 in, 2 out]
                                }
                                frame #1 {
                                n2516 = Multiply(x="Wait Before Save (s)", y=u32 1000 ("x")) -> (x*y=w3836:u32)
                                n2517 = Wait (ms)(milliseconds to wait=w3836) -> ()  [unwired: 1 out]
                                }
                                frame #2 {
                                n2518 = property on="Start Saving" class="Bool (strict)"("Value"=TRUE ("Start Saving")) -> ()  [unwired: 2 in, 2 out]
                                n2519 = case shown="\"4\"" w3838 {
                                frame Default {
                                }
                                frame "4" {
                                n2520 = property on="Fl. Triggered..." class="Bool (strict)"("Val(Sgnl)"=TRUE ("Value (Signaling)")) -> ()  [unwired: 2 in, 2 out]
                                }
                                }
                                }
                                }
                                }
                                frame "5", "6" {
                                n2521 = stacked-sequence {
                                tunnel: w3841 -> [_ _ _ _ _ _ w3853]
                                frame #0 {
                                n2522 = Replace Array Subset(array=u32[] [0] ("Index Values"), new element="Raster Set Upon Tether", index=0) -> (w3842:u32[])
                                n2523 = property on="Saved AOD Raster Scan Parameter Sets" class="Arr (strict)"("Index Values"=w3842) -> ()  [unwired: 2 in, 2 out]
                                }
                                frame #1 {
                                n2524 = Wait (ms)(milliseconds to wait=u32 500) -> ()  [unwired: 1 out]
                                }
                                frame #2 {
                                n2525 = property on="Load parameters" class="Bool (strict)"("Val(Sgnl)"=TRUE ("Value (Signaling)")) -> ()  [unwired: 2 in, 2 out]
                                n2526 = case shown="True" "Green ON During Raster" {
                                frame False {
                                }
                                frame True {
                                n2527 = property on="Green Laser ON" class="Bool (strict)"("Val(Sgnl)"=TRUE ("Value (Signaling)")) -> ()  [unwired: 2 in, 2 out]
                                }
                                }
                                }
                                frame #3 {
                                n2528 = Wait (ms)(milliseconds to wait=u32 500) -> ()  [unwired: 1 out]
                                }
                                frame #4 {
                                n2529 = property on="Trap Raster Scan" class="Bool (strict)"("Val(Sgnl)"=TRUE ("Value (Signaling)")) -> ()  [unwired: 2 in, 2 out]
                                }
                                frame #5 {
                                n2530 = Wait (ms)(milliseconds to wait=u32 2000) -> ()  [unwired: 1 out]
                                }
                                frame #6 {
                                n2531 = flat-sequence {
                                tunnel: w3853 -> [w3860]
                                frame #0 {
                                n2532 = while {
                                stop <- w3856 stop-if-true
                                n2533 = local read "Raster Scanning..."() -> (w3855:bool)
                                n2534 = local read "Saving..."() -> (w3858:bool)
                                n2535 = Wait (ms)(milliseconds to wait=u32 100) -> ()  [unwired: 1 out]
                                n2536 = Not(x=w3858) -> (.not. x?=w3857:bool)
                                n2537 = Not(x=w3855) -> (.not. x?=w3854:bool)
                                n2538 = And(x=w3857, y=w3854) -> (x .and. y?=w3856:bool)
                                }
                                }
                                frame #1 {
                                n2539 = local read "Tether"() -> (w3861:bool)
                                n2540 = case shown="True" w3861 {
                                tunnel: w3860 -> [_ w3863]
                                frame False {
                                n2541 = property on="Fish for Tether" class="Bool (strict)"("Val(Sgnl)"="Fish again after \nraster break?") -> ()  [unwired: 2 in, 2 out]
                                }
                                frame True {
                                n2542 = stacked-sequence {
                                tunnel: w3863 -> [_ w3867 _ _]
                                frame #0 {
                                n2543 = property on="Trap Delta (MHz)" class="DigNum (strict)"("Val(Sgnl)"="Move to Delta 2 (MHz)") -> ()  [unwired: 2 in, 2 out]
                                n2544 = case shown="True" "Flow ON after\ntether testing?" {
                                frame False {
                                }
                                frame True {
                                n2545 = property on="Sample Channel\nFlow" class="Bool (strict)"("Val(Sgnl)"=TRUE ("Value (Signaling)")) -> ()  [unwired: 2 in, 2 out]
                                }
                                }
                                }
                                frame #1 {
                                n2546 = flat-sequence {
                                tunnel: w3867 -> [w3869]
                                frame #0 {
                                n2547 = Wait (ms)(milliseconds to wait=u32 500) -> ()  [unwired: 1 out]
                                }
                                frame #1 {
                                n2548 = case shown="\"6\"" w3869 {
                                frame Default {
                                }
                                frame "6" {
                                n2549 = property on="Green Laser ON" class="Bool (strict)"("Val(Sgnl)"=TRUE ("Green Laser ON/Interlacing")) -> ()  [unwired: 2 in, 2 out]
                                }
                                }
                                }
                                frame #2 {
                                n2550 = Wait (ms)(milliseconds to wait=u32 500) -> ()  [unwired: 1 out]
                                }
                                frame #3 {
                                n2551 = local write "Start Saving"("Save at end (5, 6)") -> ()
                                }
                                }
                                }
                                frame #2 {
                                n2552 = local read "Bead Sep. Int. Time (s)"() -> (w3875:dbl)
                                n2553 = Multiply(x=w3875, y=1000.0) -> (x*y=w3874:dbl)
                                n2554 = Wait (ms)(milliseconds to wait=w3874) -> ()  [unwired: 1 out]
                                }
                                frame #3 {
                                n2555 = property on="Remove Offset" class="Bool (strict)"("Val(Sgnl)"=TRUE ("Value (Signaling)")) -> ()  [unwired: 2 in, 2 out]
                                }
                                }
                                }
                                }
                                }
                                }
                                }
                                }
                                }
                                frame "2", Default {
                                }
                              }
                            }
                          }
                        }
                      }
                      "Tether" <- "Tether Alarm?"
                    }
                  }
                }
                frame #2 {
                  n2556 = local read "Oscillate Set 1"() -> (w3882:bool)
                  n2557 = local read "Stop All"() -> (w3880:bool)
                  n2558 = Or(x=w3882, y=w3877) -> (x .or. y?=w3879:bool)
                  n2559 = Not(x=w3879) -> (.not. x?=w3881:bool)
                  n2560 = Compound Arithmetic op=OR(w3880, w3881) -> (w3878:bool)
                }
              }
              n2561 = node-c288() -> ()  [unwired: 2 out]
            }
            n2562 = node-c288(w3712) -> ()  [unwired: 1 out]
          }
        }
      }
      event "Fl. Triggered...": Value Change {
        n2563 = event-data() -> ()  [unwired: 7 out]
        n2564 = case shown="True" "Fl. Triggered..." {
          frame False {
          }
          frame True {
            n2565 = node-c288() -> (w3893:T35)  [unwired: 4 out]
            n2566 = timed-loop {
              timing: w3893 -> [_]
              timing-out: [_] -> w3892
              tunnel: "Action" -> [w3901]
              shift-right: [w3898] -> _
              shift-left: u8 255 -> [w3900]
              shift-right: [w3895] -> _
              shift-left: 255 -> [w3897]
              stop <- w3894 stop-if-true
              # "Reset confocal spot"
              n2567 = node-c288() -> ()  [unwired: 2 out]
              n2568 = flat-sequence {
                tunnel: w3901 -> [w3921]
                tunnel: w3900 -> [w3920]
                tunnel: [w3919] -> w3899
                tunnel: w3897 -> [w3906]
                tunnel: [w3905] -> w3896
                tunnel: [w4300] -> w3894
                tunnel: w3899 -> [w4299]
                tunnel: [w4299] -> w3898
                tunnel: [w4298] -> w3895
                tunnel: w3896 -> [w4298]
                frame #0 {
                  n2569 = local read "Delta Fl. 2"() -> (w3918:dbl)
                  n2570 = local read "Delta Fl. 1"() -> (w3913:dbl)
                  n2571 = Multiply(x="Fl. Delta Thresh. (kHz)", y=1000.0) -> (x*y=w3908:dbl)
                  n2572 = Select(t=w3913, s="APD to Watch", f=w3918) -> (s? t:f=w3909:dbl)
                  n2573 = Greater?(x=w3909, y=w3908) -> (0:w3914:bool)
                  n2574 = Or(x="Force Yank", y=w3914) -> (x .or. y?=w3912:bool)
                  n2575 = And(x=w3912, y="Yank when?") -> (x .and. y?=w3910:bool)
                  n2576 = case shown="True" w3910 {
                    tunnel: w3921 -> [w3924 w4125]
                    tunnel: w3920 -> [w3926 w4121]
                    tunnel: [w3926 w4119] -> w3919
                    tunnel: w3909 -> [w3932 _]
                    tunnel: w3908 -> [w3931 _]
                    tunnel: "Force Yank" -> [w3929 _]
                    tunnel: w3906 -> [w3928 w4118]
                    tunnel: [w3927 w4118] -> w3905
                    frame False {
                      n2577 = Negate(x=w3931) -> (-x=w3923:dbl)
                      n2578 = local write "Fl. High"(TRUE ("Fl. High")) -> ()
                      n2579 = Less?(x=w3932, y=w3923) -> (x < y?=w3930:bool)
                      n2580 = Or(x=w3929, y=w3930) -> (x .or. y?=w3925:bool)
                      n2581 = case shown="True" w3925 {
                        tunnel: w3928 -> [w3933 w3943]
                        tunnel: [w3933 w3942] -> w3927
                        tunnel: w3924 -> [_ w3941]
                        frame False {
                        }
                        frame True {
                          n2582 = flat-sequence {
                            tunnel: w3943 -> [w3949]
                            tunnel: w3941 -> [w3946]
                            tunnel: [w3948] -> w3940
